vi "总磷总氮质控流程.vi"(0 "队列输入TP":refnum<queue>, 5 "总氮量程切换":enum32{"H", "L", "AUTO"}(ring)=enum."AUTO", 7 "总磷量程切换":enum32{"H", "L", "AUTO"}(ring)=enum."AUTO", 9 "总磷":bool, 11 "总氮":bool) -> (4 "布尔":bool, 6 "总磷中断报警":bool, 8 "总氮中断报警":bool)   [LabVIEW 2016, in "质控单元.lvlib"]
panel:
  out "总磷":bool
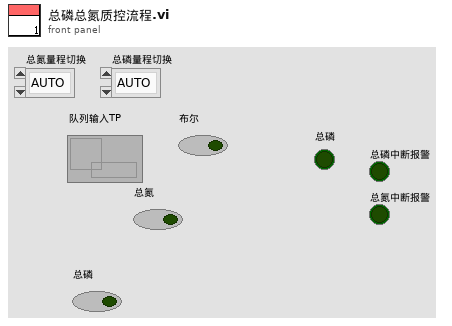
[diagram p1: front panel]
types:
  T1 = enum16{"待机", "启动氨氮水样", "氨氮测量中", "启动氨氮加标", "启动氨氮加标回收", "氨氮加标回收测量中", "启动总氮水样", "总氮测量中", "启动总氮加标", "启动总氮加标回收", "总氮加标回收测量中", "启动总磷水样", "总磷水样测量中", "启动总磷加标", "启动总磷加标回收", "总磷加标回收测量中", "结束"}
  T2 = cluster{"站号":u16, "量程切换":enum32{"H", "L", "AUTO"}, "控制命令":enum16{"启动测量", "标样核查", "零点核查", "跨度核查", "空白测试", "平行样测试", "加标回收", "空白校准", "标样校准", "初始化（清洗）", "停止测试", "仪器重启", "校时", "模式设置", "测量间隔设置"}, "模式设置":enum16{"待机", "连续模式", "周期模式", "定点模式", "受控模式", "手动模式"}, "测量间隔":u16}
  T3 = cluster{"时间标识":timestamp, "设备":string, "日志信息":string}
  T4 = cluster{"系统时间":timestamp, "工作状态":enum16{"空闲", "水样测试", "标样核查", "零点核查", "跨度核查", "空白测试", "平行样测试", "加标回收", "空白校准", "标样校准", "初始化（清洗）"}, "测量模式":enum16{"待机", "连续模式", "周期模式", "定点模式", "受控模式", "手动模式"}, "告警代码":enum16{"无告警", "缺试剂告警", "缺水样告警", "缺蒸馏水告警", "缺标液告警", "仪表漏液告警", "标定异常告警", "超量程告警", "加热异常", "低试剂预警", "超上限告警", "超下限告警", "仪表内部其他异常", "滴定异常告警", "电极异常告警", "量程切换告警", "参数设置告警", "PH电极电位异常", "电导率电极异常", "浊度光度异常", "溶解氧电极异常", "溶解氧光强异常", "温度异常告警", "PH异常告警", "溶解氧异常告警", "电导率异常告警", "浊度异常告警", "叶绿素异常告警", "藻密度异常告警", "蓝绿藻异常告警", "ORP异常告警", "氨氮异常告警", "清洁刷异常告警", "SD卡异常告警", "蓝牙异常告警", "Wifi异常告警", "流程异常告警"}, "故障代码":enum16{"无故障", "电机故障", "温度故障", "通讯故障", "滴定故障"}, "日志代码":u16, "软件版本":u16, "F0":sgl, "F1":sgl, "F2":sgl, "F3":sgl, "T":sgl, "H":sgl, "id":u16, "flowid":u16, "量程":u16, "总磷控温温度1":sgl, "营养盐控温温度2":sgl, "ADC":sgl}
  T5 = enum16{"空闲", "水样测试", "标样核查", "零点核查", "跨度核查", "空白测试", "平行样测试", "加标回收", "空白校准", "标样校准", "初始化（清洗）"}
  T6 = cluster{"因子编码":u32, "单位":u16, "标样参考值":sgl, "水样数据时间":timestamp, "水样实测值":sgl, "水样数据标识":string, "标样数据时间":timestamp, "标样实测值":sgl, "标样数据标识":string, "空白数据时间":timestamp, "空白实测值":sgl, "空白数据标识":string, "零点核查数据时间":timestamp, "零点核查实测值":sgl, "零点核查数据标识":string, "跨度核查数据时间":timestamp, "跨度核查实测值":sgl, "跨度核查数据标识":string, "加标回收数据时间":timestamp, "加标回收实测值":sgl, "加标回收数据标识":string, "平行样数据时间":timestamp, "平行样实测值":sgl, "平行样数据标识":string}
  T7 = cluster{"量程":dbl, "检出限":dbl, "加标前水样浓度":dbl, "加标后水样浓度":dbl, "加标水杯定容体积":dbl, "加标母液浓度":dbl, "加标体积":dbl, "加标回收率":dbl}
  T8 = cluster{"氨氮":u8, "总磷":u8, "总氮":u8, "CODMn":u8, "CODCr":u8}
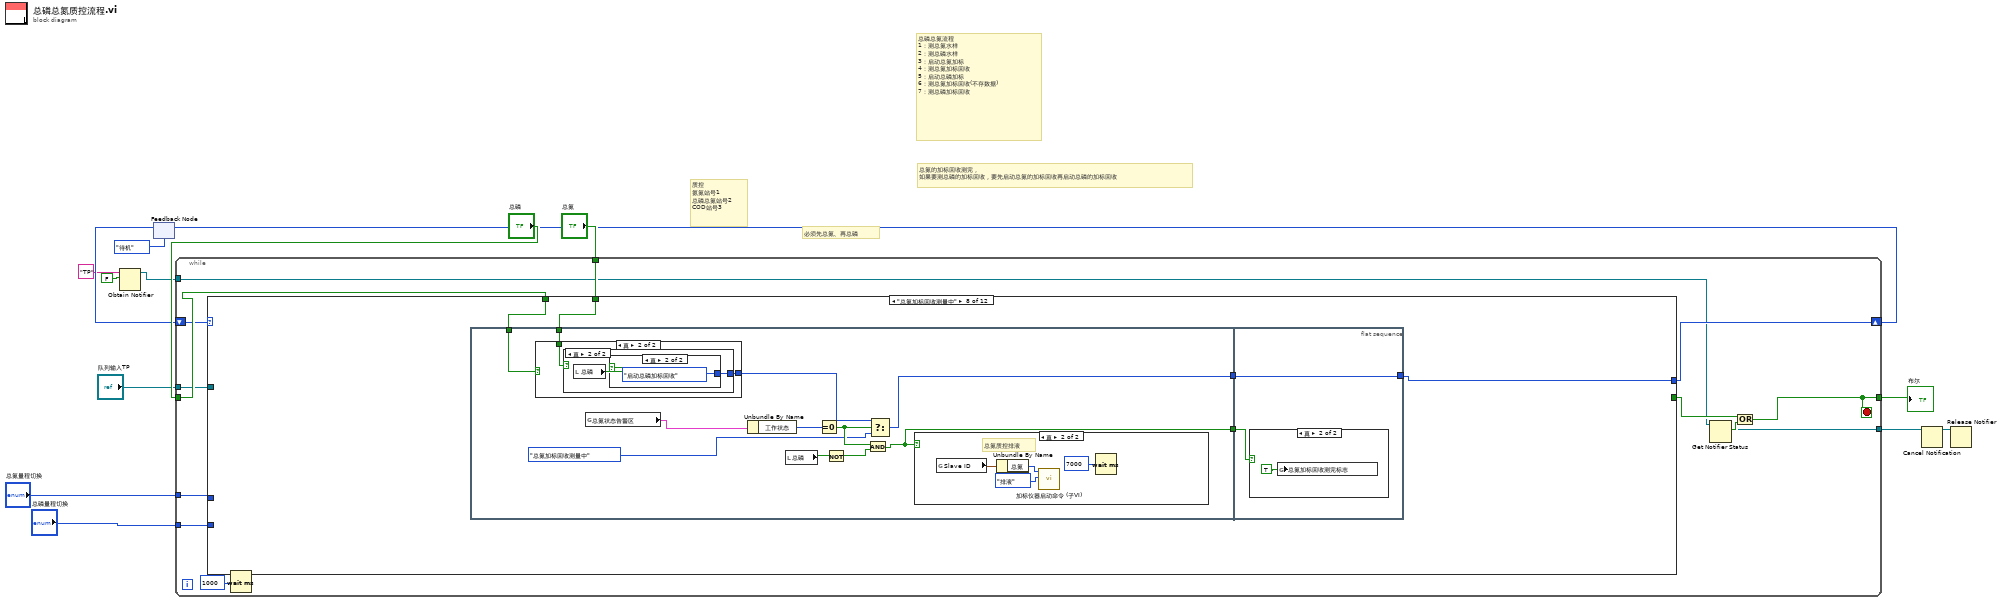
[diagram p0: block diagram]
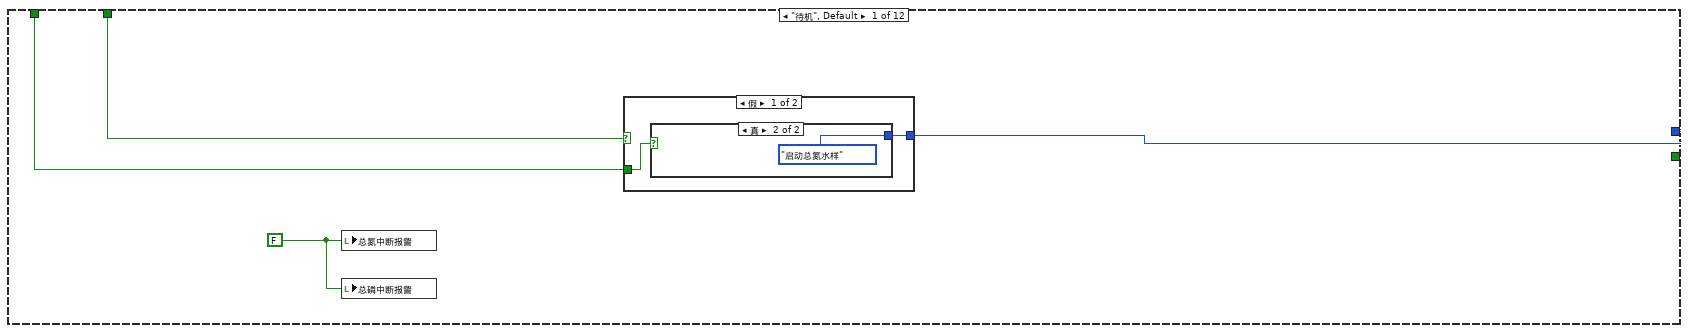
[diagram p2: hidden frame]
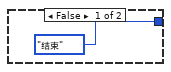
[diagram p3: hidden frame]
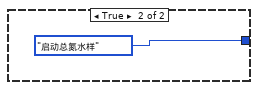
[diagram p4: hidden frame]
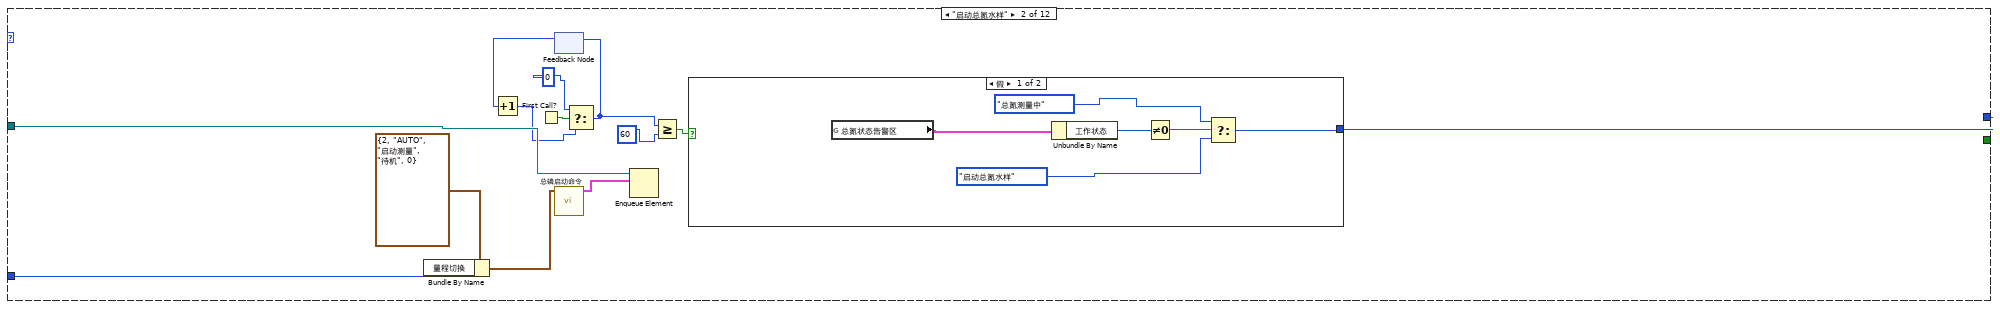
[diagram p5: hidden frame]
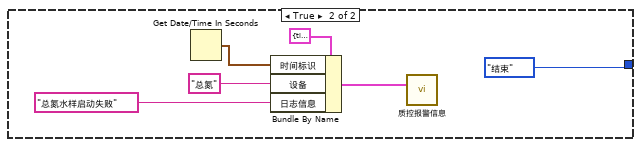
[diagram p6: hidden frame]
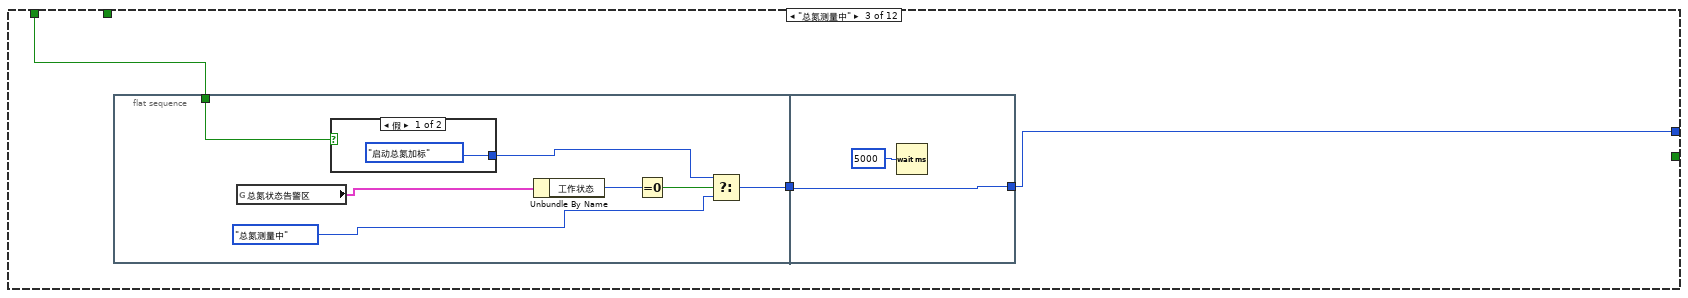
[diagram p7: hidden frame]
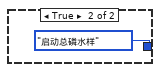
[diagram p8: hidden frame]
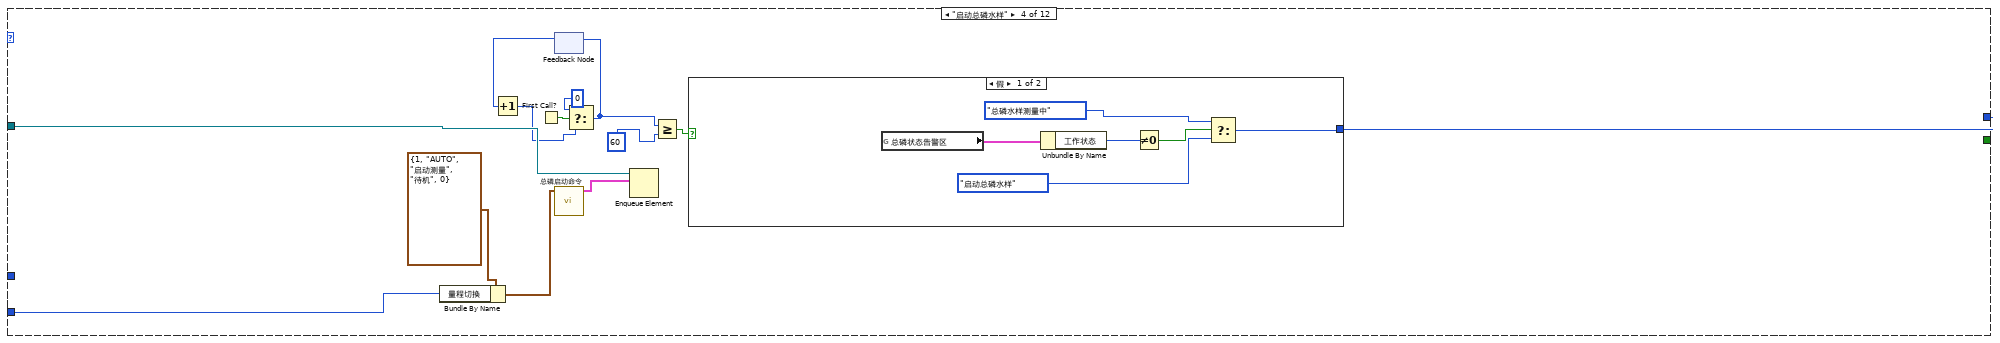
[diagram p9: hidden frame]
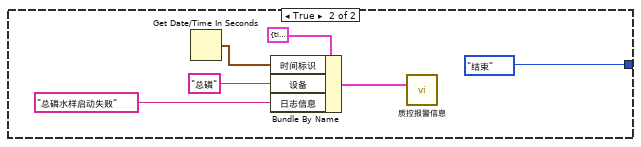
[diagram p10: hidden frame]
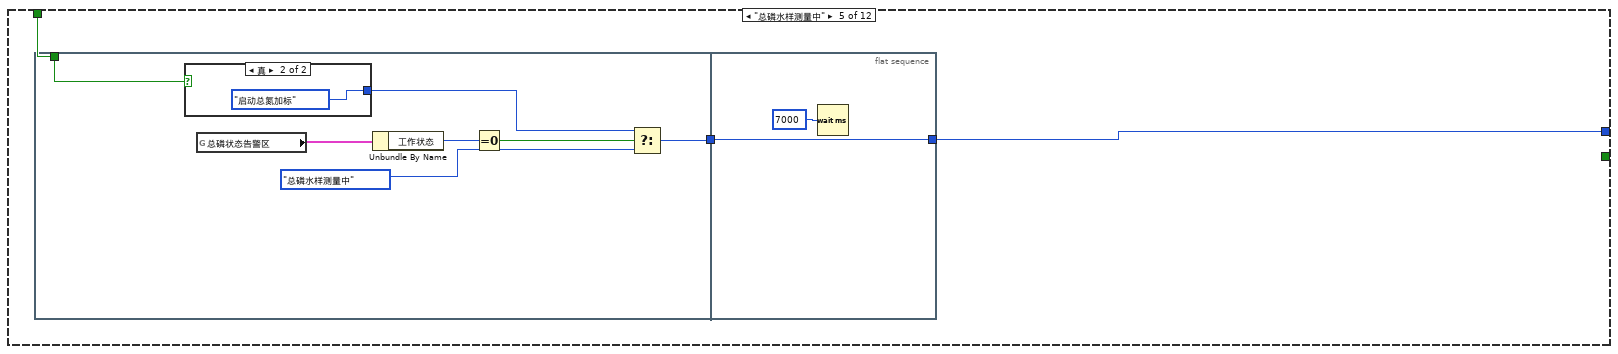
[diagram p11: hidden frame]
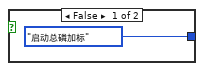
[diagram p12: hidden frame]
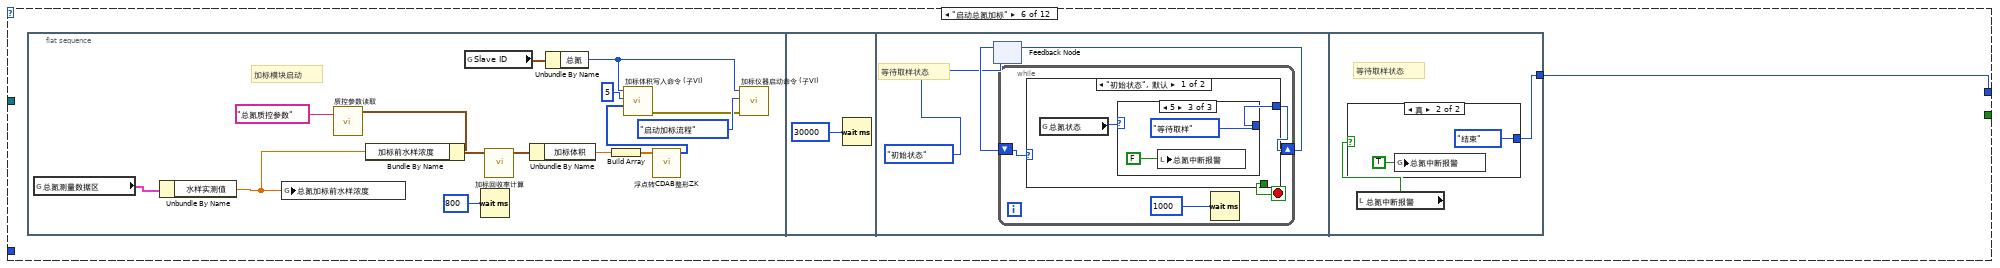
[diagram p13: hidden frame]
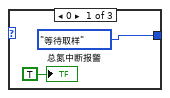
[diagram p14: hidden frame]
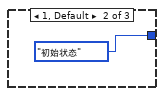
[diagram p15: hidden frame]
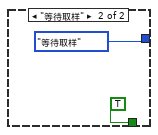
[diagram p16: hidden frame]
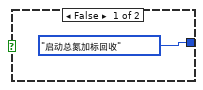
[diagram p17: hidden frame]
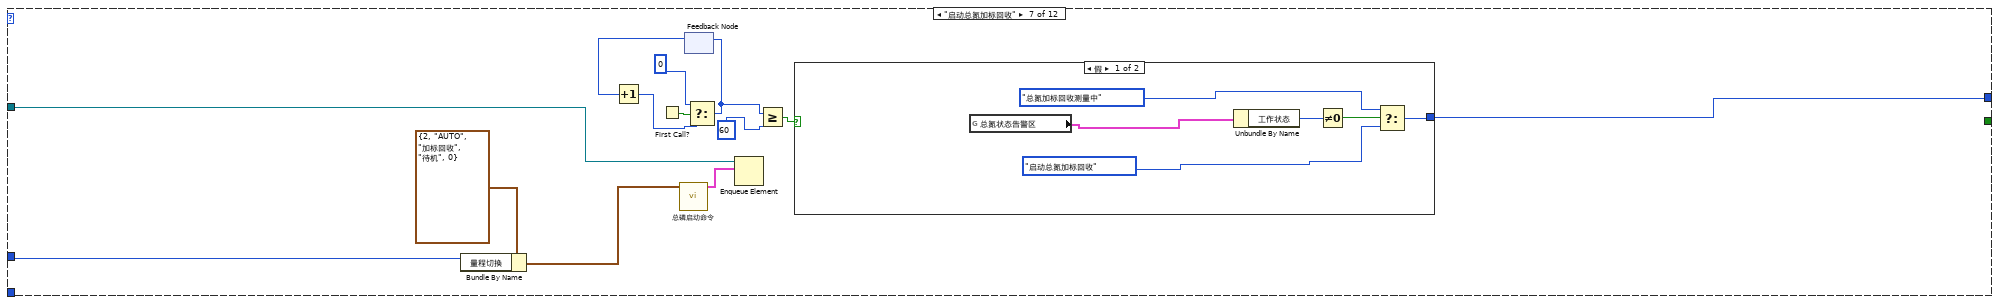
[diagram p18: hidden frame]
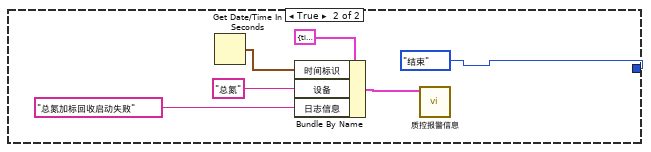
[diagram p19: hidden frame]
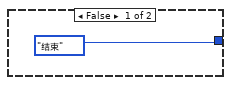
[diagram p20: hidden frame]
diagram:
  # "总磷总氮流程\n1：测总氮水样\n2：测总磷水样\n3：启动总氮加标\n4：测总氮加标回收\n5：启动总磷加标\n6：测总氮加标回收(不存数据)\n7：测总磷加标回收"
  # "总氮的加标回收测完，\n如果要测总磷的加标回收，要先启动总氮的加标回收再启动总磷的加标回收"
  # "质控\n氨氮站号1   \n总磷总氮站号2\nCOD站号3"
  # "必须先总氮、再总磷"
  n1 = Obtain Notifier(name (unnamed)="TP" ("名称（未命名）"), notification data type=FALSE) -> (notifier out=w3:refnum<notifier>)  [unwired: 2 in, 2 out]
  n2 = feedback #1(T1."待机") -> (w6:T1)
  n3 = while {
    tunnel: "队列输入TP" -> [w26]
    tunnel: "总氮" -> [w25]
    tunnel: "总氮量程切换" -> [w23]
    tunnel: "总磷量程切换" -> [w22]
    shift-right: [w24] -> w9
    shift-left: w6 -> [w21]
    tunnel: "总磷" -> [w27]
    tunnel: [w17] -> w13
    tunnel: w3 -> [w16]
    tunnel: [w15] -> w1
    stop <- w17 stop-if-true
    n4 = case shown="\"总氮加标回收测量中\"" w21 {
      tunnel: [w31 w48 w63 w87 w103 w115 w156 w180 w209 w253 w276 T1."结束"] -> w24
      tunnel: w26 -> [_ w49 _ w88 _ _ w158 _ _ w254 _ _]
      tunnel: [_ _ _ _ _ _ _ _ _ _ _ TRUE] -> w18
      tunnel: w27 -> [w30 _ w62 _ _ _ _ w181 _ _ _ _]
      tunnel: w25 -> [w29 _ _ _ w101 _ _ w179 _ _ _ _]
      tunnel: w23 -> [_ w37 _ _ _ _ w153 _ _ _ _ _]
      tunnel: w22 -> [_ _ _ w76 _ _ _ _ _ w249 _ _]
      frame "待机", Default {
        w28 = FALSE ("总氮中断报警")
        n5 = local write "总氮中断报警"(w28) -> ()
        n6 = local write "总磷中断报警"(w28) -> ()
        n7 = case shown="假" w29 {
          tunnel: w30 -> [w32 _]
          tunnel: [w33 T1."启动总氮水样"] -> w31
          frame False {
            n8 = case shown="真" w32 {
              tunnel: [T1."结束" T1."启动总氮水样"] -> w33
              frame False {
              }
              frame True {
              }
            }
          }
          frame True {
          }
        }
      }
      frame "启动总氮水样" {
        n9 = Bundle By Name(cluster=T2 {"站号"=2, "量程切换"=enum."AUTO", "控制命令"=enum."启动测量", "模式设置"=enum."待机", "测量间隔"=0} ("参数"), "量程切换"=w37) -> (w38:T2)
        n10 = First Call?() -> (First Call?: T/F=w46:bool)
        n11 = feedback #2() -> (w45:i32)  [unwired: 1 in]
        n12 = Increment(x=w45) -> (x+1=w44:i32)
        n13 = call "总磷启动命令.vi"("参数"=w38) -> ("启动命令"=w40:cluster{"命令":string, "data":variant})  [unwired: 10 in]
        n14 = Select(t=0, s=w46, f=w44) -> (s? t:f=w43:i32)
        n15 = feedback-in #2(w43) -> ()
        n16 = Enqueue Element(queue=w49, element=w40) -> ()  [unwired: 2 in, 3 out]
        n17 = Greater Or Equal?(x=w43, y=60) -> (x >= y?=w41:bool)
        n18 = case shown="假" w41 {
          tunnel: [w53 T1."结束"] -> w48
          frame False {
            n19 = global read "与总氮交互全局.vi" "总氮状态告警区"() -> (w50:T4)
            n20 = Unbundle By Name(w50) -> ("工作状态"=w54:T5)
            n21 = Not Equal To 0?(x=w54) -> (x != 0?=w55:bool)
            n22 = Select(t=T1."总氮测量中", s=w55, f=T1."启动总氮水样") -> (s? t:f=w53:T1)
          }
          frame True {
            n23 = Get Date/Time In Seconds() -> (seconds since 1Jan1904=w61:timestamp)
            n24 = Bundle By Name(cluster=T3 {"时间标识"=timestamp(0 s since 1904-01-01), "设备"="", "日志信息"=""} ("data in"), "时间标识"=w61, "设备"="总氮", "日志信息"="总氮水样启动失败") -> (w57:T3)
            n25 = call "质控报警信息.vi"("data in"=w57) -> ()  [unwired: 10 in, 1 out]
          }
        }
      }
      frame "总氮测量中" {
        n26 = flat-sequence {
          tunnel: [w70] -> w64
          tunnel: w62 -> [w66]
          tunnel: [w75] -> w63
          tunnel: w64 -> [w75]
          frame #0 {
            n27 = global read "与总氮交互全局.vi" "总氮状态告警区"() -> (w65:T4)
            n28 = case shown="假" w66 {
              tunnel: [T1."启动总氮加标" T1."启动总磷水样"] -> w68
              frame False {
              }
              frame True {
              }
            }
            n29 = Unbundle By Name(w65) -> ("工作状态"=w71:T5)
            n30 = Equal To 0?(x=w71) -> (x = 0?=w69:bool)
            n31 = Select(t=w68, s=w69, f=T1."总氮测量中") -> (s? t:f=w70:T1)
          }
          frame #1 {
            n32 = Wait (ms)(milliseconds to wait=u32 5000 ("等待时间（毫秒）")) -> ()  [unwired: 1 out]
          }
        }
      }
      frame "启动总磷水样" {
        n33 = Bundle By Name(cluster=T2 {"站号"=1, "量程切换"=enum."AUTO", "控制命令"=enum."启动测量", "模式设置"=enum."待机", "测量间隔"=0} ("参数"), "量程切换"=w76) -> (w77:T2)
        n34 = First Call?() -> (First Call?: T/F=w85:bool)
        n35 = feedback #3() -> (w84:i32)  [unwired: 1 in]
        n36 = Increment(x=w84) -> (x+1=w83:i32)
        n37 = call "总磷启动命令.vi"("参数"=w77) -> ("启动命令"=w79:cluster{"命令":string, "data":variant})  [unwired: 10 in]
        n38 = Select(t=0, s=w85, f=w83) -> (s? t:f=w82:i32)
        n39 = feedback-in #3(w82) -> ()
        n40 = Enqueue Element(queue=w88, element=w79) -> ()  [unwired: 2 in, 3 out]
        n41 = Greater Or Equal?(x=w82, y=60) -> (x >= y?=w80:bool)
        n42 = case shown="假" w80 {
          tunnel: [w91 T1."结束"] -> w87
          frame False {
            n43 = global read "与总磷交互全局.vi" "总磷状态告警区"() -> (w92:T4)
            n44 = Unbundle By Name(w92) -> ("工作状态"=w93:T5)
            n45 = Not Equal To 0?(x=w93) -> (x != 0?=w94:bool)
            n46 = Select(t=T1."总磷水样测量中", s=w94, f=T1."启动总磷水样") -> (s? t:f=w91:T1)
          }
          frame True {
            n47 = Get Date/Time In Seconds() -> (seconds since 1Jan1904=w100:timestamp)
            n48 = Bundle By Name(cluster=T3 {"时间标识"=timestamp(0 s since 1904-01-01), "设备"="", "日志信息"=""} ("data in"), "时间标识"=w100, "设备"="总磷", "日志信息"="总磷水样启动失败") -> (w96:T3)
            n49 = call "质控报警信息.vi"("data in"=w96) -> ()  [unwired: 10 in, 1 out]
          }
        }
      }
      frame "总磷水样测量中" {
        n50 = flat-sequence {
          tunnel: [w108] -> w102
          tunnel: w101 -> [w105]
          tunnel: [w114] -> w103
          tunnel: w102 -> [w114]
          frame #0 {
            n51 = case shown="真" w105 {
              tunnel: [T1."启动总磷加标" T1."启动总氮加标"] -> w106
              frame False {
              }
              frame True {
              }
            }
            n52 = global read "与总磷交互全局.vi" "总磷状态告警区"() -> (w109:T4)
            n53 = Unbundle By Name(w109) -> ("工作状态"=w110:T5)
            n54 = Equal To 0?(x=w110) -> (x = 0?=w107:bool)
            n55 = Select(t=w106, s=w107, f=T1."总磷水样测量中") -> (s? t:f=w108:T1)
          }
          frame #1 {
            n56 = Wait (ms)(milliseconds to wait=u32 7000 ("等待时间（毫秒）")) -> ()  [unwired: 1 out]
          }
        }
      }
      frame "启动总氮加标" {
        n57 = flat-sequence {
          tunnel: [w149] -> w115
          frame #0 {
            # "加标模块启动"
            n58 = global read "与总氮交互全局.vi" "总氮测量数据区"() -> (w122:T6)
            n59 = Unbundle By Name(w122) -> ("水样实测值"=w123:sgl)
            n60 = global write "水样浓度全局.vi" "总氮加标前水样浓度"(w123) -> ()
            n61 = call "质控参数读取.vi"("section"="总氮质控参数") -> ("参数"=w125:T7)  [unwired: 9 in, 1 out]
            n62 = Bundle By Name(cluster=w125, "加标前水样浓度"=w123) -> (w129:T7)
            n63 = global read "断电保存全局.vi" "Slave ID"() -> (w120:T8)
            n64 = Wait (ms)(milliseconds to wait=u32 800 ("等待时间（毫秒）")) -> ()  [unwired: 1 out]
            n65 = call "加标回收率计算.vi"("参数"=w129) -> ("参数 out"=w128:T7)  [unwired: 9 in, 1 out]
            n66 = Unbundle By Name(w128) -> ("加标体积"=w126:dbl)
            n67 = Unbundle By Name(w120) -> ("总氮"=w121:u8)
            n68 = Build Array(w126) -> (w127:dbl[])
            n69 = call "浮点转CDAB整形ZK.vi"("浮点数"=w127) -> ("CDAB整形输出"=w116:u16[])  [unwired: 10 in]
            n70 = call "加标体积写入命令 (子VI).vi"("values"=w116, "starting address"=u16 5, "Slave ID"=w121) -> ("错误输出"=w118:errorcluster)  [unwired: 8 in]
            n71 = call "加标仪器启动命令 (子VI).vi"("错误输入（无错误）"=w118, "启动命令"=enum16{"启动水样流程", "启动加标流程", "排液", "停止"}."启动加标流程", "仪器"=w121) -> ()  [unwired: 8 in, 1 out]
          }
          frame #1 {
            n72 = Wait (ms)(milliseconds to wait=u32 30000 ("等待时间（毫秒）")) -> ()  [unwired: 1 out]
          }
          frame #2 {
            # "等待取样状态"
            n73 = feedback #4(enum16{"初始状态", "等待取样"}."初始状态") -> (w134:enum16{"初始状态", "等待取样"})
            n74 = while {
              shift-right: [w137] -> w133
              shift-left: w134 -> [w138]
              stop <- w136 stop-if-true
              n75 = case shown="\"初始状态\", 默认" w138 {
                tunnel: [w140 enum16{"初始状态", "等待取样"}."等待取样"] -> w137
                tunnel: [_ TRUE] -> w136
                frame "初始状态", Default {
                  n76 = global read "加标回收状态全局变量.vi" "总氮状态"() -> (w139:u16)
                  n77 = case shown="5" w139 {
                    tunnel: [enum16{"初始状态", "等待取样"}."等待取样" enum16{"初始状态", "等待取样"}."初始状态" enum16{"初始状态", "等待取样"}."等待取样"] -> w140
                    frame 0 {
                      "总氮中断报警" <- TRUE ("总氮中断报警")
                    }
                    frame 1, Default {
                    }
                    frame 5 {
                      n78 = local write "总氮中断报警"(FALSE ("总氮中断报警")) -> ()
                    }
                  }
                }
                frame "等待取样" {
                }
              }
              n79 = Wait (ms)(milliseconds to wait=u32 1000 ("等待时间（毫秒）")) -> ()  [unwired: 1 out]
            }
            n80 = feedback-in #4(w133) -> ()
          }
          frame #3 {
            # "等待取样状态"
            n81 = local read "总氮中断报警"() -> (w148:bool)
            n82 = case shown="真" w148 {
              tunnel: [T1."启动总氮加标回收" T1."结束"] -> w149
              frame False {
              }
              frame True {
                n83 = global write "质控中断报警全局.vi" "总氮中断报警"(TRUE ("总氮中断报警")) -> ()
              }
            }
          }
        }
      }
      frame "启动总氮加标回收" {
        n84 = Bundle By Name(cluster=T2 {"站号"=2, "量程切换"=enum."AUTO", "控制命令"=enum."加标回收", "模式设置"=enum."待机", "测量间隔"=0} ("参数"), "量程切换"=w153) -> (w154:T2)
        n85 = First Call?() -> (First Call?: T/F=w164:bool)
        n86 = call "总磷启动命令.vi"("参数"=w154) -> ("启动命令"=w157:cluster{"命令":string, "data":variant})  [unwired: 10 in]
        n87 = feedback #5() -> (w163:i32)  [unwired: 1 in]
        n88 = Increment(x=w163) -> (x+1=w162:i32)
        n89 = Select(t=0, s=w164, f=w162) -> (s? t:f=w161:i32)
        n90 = feedback-in #5(w161) -> ()
        n91 = Enqueue Element(queue=w158, element=w157) -> ()  [unwired: 2 in, 3 out]
        n92 = Greater Or Equal?(x=w161, y=60) -> (x >= y?=w159:bool)
        n93 = case shown="假" w159 {
          tunnel: [w169 T1."结束"] -> w156
          frame False {
            n94 = global read "与总氮交互全局.vi" "总氮状态告警区"() -> (w166:T4)
            n95 = Unbundle By Name(w166) -> ("工作状态"=w171:T5)
            n96 = Not Equal To 0?(x=w171) -> (x != 0?=w170:bool)
            n97 = Select(t=T1."总氮加标回收测量中", s=w170, f=T1."启动总氮加标回收") -> (s? t:f=w169:T1)
          }
          frame True {
            n98 = Get Date/Time In Seconds() -> (seconds since 1Jan1904=w177:timestamp)
            n99 = Bundle By Name(cluster=T3 {"时间标识"=timestamp(0 s since 1904-01-01), "设备"="", "日志信息"=""} ("data in"), "时间标识"=w177, "设备"="总氮", "日志信息"="总氮加标回收启动失败") -> (w173:T3)
            n100 = call "质控报警信息.vi"("data in"=w173) -> ()  [unwired: 10 in, 1 out]
          }
        }
      }
      frame "总氮加标回收测量中" {
        n101 = flat-sequence {
          tunnel: [w192] -> w182
          tunnel: w181 -> [w189]
          tunnel: w179 -> [w185]
          tunnel: [w183] -> w178
          tunnel: [w207] -> w180
          tunnel: w182 -> [w207]
          tunnel: w178 -> [w206]
          frame #0 {
            n102 = case shown="真" w189 {
              tunnel: [T1."结束" w196] -> w191
              tunnel: w185 -> [_ w195]
              frame False {
              }
              frame True {
                n103 = case shown="真" w195 {
                  tunnel: [T1."启动总磷加标回收" w199] -> w196
                  frame False {
                  }
                  frame True {
                    n104 = local read "总磷"() -> (w198:bool)
                    n105 = case shown="真" w198 {
                      tunnel: [T1."启动总磷加标" T1."启动总磷加标回收"] -> w199
                      frame False {
                      }
                      frame True {
                      }
                    }
                  }
                }
              }
            }
            n106 = global read "与总氮交互全局.vi" "总氮状态告警区"() -> (w184:T4)
            n107 = Unbundle By Name(w184) -> ("工作状态"=w193:T5)
            n108 = local read "总磷"() -> (w187:bool)
            n109 = Equal To 0?(x=w193) -> (x = 0?=w190:bool)
            n110 = Not(x=w187) -> (.not. x?=w186:bool)
            n111 = And(x=w190, y=w186) -> (x .and. y?=w183:bool)
            n112 = Select(t=w191, s=w190, f=T1."总氮加标回收测量中") -> (s? t:f=w192:T1)
            n113 = case shown="真" w183 {
              frame False {
              }
              frame True {
                # "总氮质控排液"
                n114 = global read "断电保存全局.vi" "Slave ID"() -> (w203:T8)
                n115 = Unbundle By Name(w203) -> ("总氮"=w204:u8)
                n116 = call "加标仪器启动命令 (子VI).vi"("启动命令"=enum16{"启动水样流程", "启动加标流程", "排液", "停止"}."排液", "仪器"=w204) -> ()  [unwired: 9 in, 1 out]
                n117 = Wait (ms)(milliseconds to wait=u32 7000 ("等待时间（毫秒）")) -> ()  [unwired: 1 out]
              }
            }
          }
          frame #1 {
            n118 = case shown="真" w206 {
              frame False {
              }
              frame True {
                n119 = global write "质控测完标志全局 1.vi" "总氮加标回收测完标志"(TRUE) -> ()
              }
            }
          }
        }
      }
      frame "启动总磷加标" {
        n120 = flat-sequence {
          tunnel: [w245] -> w209
          frame #0 {
            n121 = Wait (ms)(milliseconds to wait=u32 180000 ("等待时间（毫秒）")) -> ()  [unwired: 1 out]
          }
          frame #1 {
            # "加标模块启动"
            n122 = global read "与总磷交互全局.vi" "总磷测量数据区"() -> (w218:T6)
            n123 = Unbundle By Name(w218) -> ("水样实测值"=w217:sgl)
            n124 = call "质控参数读取.vi"("section"="总磷质控参数") -> ("参数"=w220:T7)  [unwired: 9 in, 1 out]
            n125 = Bundle By Name(cluster=w220, "加标前水样浓度"=w217) -> (w224:T7)
            n126 = global write "水样浓度全局.vi" "总磷加标前水样浓度"(w217) -> ()
            n127 = Wait (ms)(milliseconds to wait=u32 800 ("等待时间（毫秒）")) -> ()  [unwired: 1 out]
            n128 = global read "断电保存全局.vi" "Slave ID"() -> (w215:T8)
            n129 = call "加标回收率计算.vi"("参数"=w224) -> ("参数 out"=w223:T7)  [unwired: 9 in, 1 out]
            n130 = Unbundle By Name(w223) -> ("加标体积"=w221:dbl)
            n131 = Unbundle By Name(w215) -> ("总磷"=w216:u8)
            n132 = Build Array(w221) -> (w222:dbl[])
            n133 = call "浮点转CDAB整形ZK.vi"("浮点数"=w222) -> ("CDAB整形输出"=w211:u16[])  [unwired: 10 in]
            n134 = call "加标体积写入命令 (子VI).vi"("values"=w211, "starting address"=u16 5, "Slave ID"=w216) -> ("错误输出"=w213:errorcluster)  [unwired: 8 in]
            n135 = call "加标仪器启动命令 (子VI).vi"("错误输入（无错误）"=w213, "启动命令"=enum16{"启动水样流程", "启动加标流程", "排液", "停止"}."启动加标流程", "仪器"=w216) -> ()  [unwired: 8 in, 1 out]
          }
          frame #2 {
            n136 = Wait (ms)(milliseconds to wait=u32 10000 ("等待时间（毫秒）")) -> ()  [unwired: 1 out]
          }
          frame #3 {
            # "等待取样状态"
            n137 = feedback #6(enum16{"初始状态", "等待取样"}."初始状态") -> (w229:enum16{"初始状态", "等待取样"})
            n138 = while {
              shift-right: [w232] -> w228
              shift-left: w229 -> [w233]
              stop <- w231 stop-if-true
              n139 = case shown="\"初始状态\", 默认" w233 {
                tunnel: [w235 enum16{"初始状态", "等待取样"}."等待取样"] -> w232
                tunnel: [_ TRUE] -> w231
                frame "初始状态", Default {
                  n140 = global read "加标回收状态全局变量.vi" "总磷状态"() -> (w234:u16)
                  n141 = case shown="5" w234 {
                    tunnel: [enum16{"初始状态", "等待取样"}."等待取样" enum16{"初始状态", "等待取样"}."初始状态" enum16{"初始状态", "等待取样"}."等待取样"] -> w235
                    frame 0 {
                      "总磷中断报警" <- TRUE ("总磷中断报警")
                    }
                    frame 1, Default {
                    }
                    frame 5 {
                      n142 = local write "总磷中断报警"(FALSE ("总磷中断报警")) -> ()
                    }
                  }
                }
                frame "等待取样" {
                  "总磷" <- TRUE
                }
              }
              n143 = Wait (ms)(milliseconds to wait=u32 1000 ("等待时间（毫秒）")) -> ()  [unwired: 1 out]
            }
            n144 = feedback-in #6(w228) -> ()
          }
          frame #4 {
            n145 = local read "总磷中断报警"() -> (w244:bool)
            n146 = case shown="真" w244 {
              tunnel: [T1."启动总氮加标回收" T1."结束"] -> w245
              frame False {
                # "等待取样状态"
              }
              frame True {
                n147 = global write "质控中断报警全局.vi" "总磷中断报警"(TRUE ("总磷中断报警")) -> ()
              }
            }
          }
        }
      }
      frame "启动总磷加标回收" {
        n148 = Bundle By Name(cluster=T2 {"站号"=1, "量程切换"=enum."AUTO", "控制命令"=enum."加标回收", "模式设置"=enum."待机", "测量间隔"=0} ("参数"), "量程切换"=w249) -> (w250:T2)
        n149 = First Call?() -> (First Call?: T/F=w261:bool)
        n150 = feedback #7() -> (w260:i32)  [unwired: 1 in]
        n151 = Increment(x=w260) -> (x+1=w259:i32)
        n152 = call "总磷启动命令.vi"("参数"=w250) -> ("启动命令"=w255:cluster{"命令":string, "data":variant})  [unwired: 10 in]
        n153 = Select(t=0, s=w261, f=w259) -> (s? t:f=w258:i32)
        n154 = feedback-in #7(w258) -> ()
        n155 = Enqueue Element(queue=w254, element=w255) -> ()  [unwired: 2 in, 3 out]
        n156 = Greater Or Equal?(x=w258, y=60) -> (x >= y?=w256:bool)
        n157 = case shown="真" w256 {
          tunnel: [w265 T1."结束"] -> w253
          frame False {
            n158 = global read "与总磷交互全局.vi" "总磷状态告警区"() -> (w266:T4)
            n159 = Unbundle By Name(w266) -> ("工作状态"=w267:T5)
            n160 = Not Equal To 0?(x=w267) -> (x != 0?=w268:bool)
            n161 = Select(t=T1."总磷加标回收测量中", s=w268, f=T1."启动总磷加标回收") -> (s? t:f=w265:T1)
          }
          frame True {
            n162 = Get Date/Time In Seconds() -> (seconds since 1Jan1904=w274:timestamp)
            n163 = Bundle By Name(cluster=T3 {"时间标识"=timestamp(0 s since 1904-01-01), "设备"="", "日志信息"=""} ("data in"), "时间标识"=w274, "设备"="总磷", "日志信息"="总磷加标回收启动失败") -> (w270:T3)
            n164 = call "质控报警信息.vi"("data in"=w270) -> ()  [unwired: 10 in, 1 out]
          }
        }
        n165 = local write "总磷"(FALSE ("总磷")) -> ()
      }
      frame "总磷加标回收测量中" {
        n166 = flat-sequence {
          tunnel: [w281] -> w277
          tunnel: [w278] -> w275
          tunnel: [w289] -> w276
          tunnel: w277 -> [w289]
          tunnel: w275 -> [w288]
          frame #0 {
            n167 = global read "与总磷交互全局.vi" "总磷状态告警区"() -> (w282:T4)
            n168 = Unbundle By Name(w282) -> ("工作状态"=w283:T5)
            n169 = Equal To 0?(x=w283) -> (x = 0?=w278:bool)
            n170 = Select(t=T1."结束", s=w278, f=T1."总磷加标回收测量中") -> (s? t:f=w281:T1)
            n171 = case shown="真" w278 {
              frame False {
              }
              frame True {
                # "总磷质控排液"
                n172 = global read "断电保存全局.vi" "Slave ID"() -> (w285:T8)
                n173 = Wait (ms)(milliseconds to wait=u32 5000 ("等待时间（毫秒）")) -> ()  [unwired: 1 out]
                n174 = Unbundle By Name(w285) -> ("总磷"=w286:u8)
                n175 = call "加标仪器启动命令 (子VI).vi"("启动命令"=enum16{"启动水样流程", "启动加标流程", "排液", "停止"}."排液", "仪器"=w286) -> ()  [unwired: 9 in, 1 out]
              }
            }
          }
          frame #1 {
            n176 = case shown="真" w288 {
              frame False {
              }
              frame True {
                n177 = global write "质控测完标志全局 1.vi" "总磷加标回收测完标志"(TRUE) -> ()
              }
            }
          }
        }
      }
      frame "结束" {
        n178 = Wait (ms)(milliseconds to wait=u32 5000 ("等待时间（毫秒）")) -> ()  [unwired: 1 out]
      }
    }
    n179 = Wait (ms)(milliseconds to wait=u32 1000 ("等待时间（毫秒）")) -> ()  [unwired: 1 out]
    n180 = Get Notifier Status(notifier=w16) -> (notifier out=w15:refnum<notifier>, current notification=w19:bool)  [unwired: 1 in, 3 out]
    n181 = Or(x=w18, y=w19) -> (x .or. y?=w17:bool)
  }
  "布尔" <- w13
  n182 = feedback-in #1(w9) -> ()
  n183 = Cancel Notification(0:w1) -> (8:w2:refnum<notifier>)  [unwired: 1 in, 2 out]
  n184 = Release Notifier(notifier=w2) -> ()  [unwired: 2 in, 3 out]
